vi "ResonanceAnalyzer_New_Guess_Frequency.vi"() -> ()   [LabVIEW 2014]
uses:
  <vilib>/imath/engines/lvmath/Plug In/_Char/NIMS_CH_character datatype.ctl
  <vilib>/imath/engines/lvmath2/RunTimeEngine/Managers/WorkSpace/UID Generator.vi
  <vilib>/imath/engines/lvmath2/RunTimeEngine/RunTimeType/NIMS_RunTimeType_From StrictType (excl LVString).vi
  <instcachedir>/0/NIMS_RunTimeType_From StrictType (excl LVString)_15A5391EEA9C4AACB9955AC755B83D29.lvgen/NIMS_RunTimeType_From StrictType (excl LVString)_15A5391EEA9C4AACB9955AC755B83D29_000.vi
  <vilib>/imath/engines/lvmath2/RunTimeEngine/LocalVariableDefStatement/MC_LocalVariableDefStatement_Display.vi
  <vilib>/imath/engines/lvmath2/RunTimeEngine/BuiltInFunctions/int32/NIMS_int32(real).vi
  <instcachedir>/0/NIMS_int32(real)_9F6AE75EF4BE45429513317A1C5A7040.lvgen/NIMS_int32(real)_9F6AE75EF4BE45429513317A1C5A7040_000.vi
  <vilib>/imath/engines/lvmath2/RunTimeEngine/BuiltInFunctions/linramp/NIMS_linramp.vi
  <vilib>/imath/engines/lvmath2/RunTimeEngine/RangeToken/NIMS_Range_R2 - Integer.vi
  <instcachedir>/0/NIMS_Range_R2 - Integer_2D1304BAF97744E0A293025746CBADFC.lvgen/NIMS_Range_R2 - Integer_2D1304BAF97744E0A293025746CBADFC_000.vi
  <vilib>/imath/engines/lvmath2/RunTimeEngine/CommandStatement/MC_CommandStatement_break.vi
  <vilib>/imath/engines/lvmath2/RunTimeEngine/IndexRead/NIMS V(S).vi
  <instcachedir>/0/NIMS V(S)_0488751826AF41519A22953C041130DC.lvgen/NIMS V(S)_0488751826AF41519A22953C041130DC_000.vi
  <vilib>/imath/engines/lvmath2/RunTimeEngine/IndexReplace/NIMS V(S)=S.vi
  <instcachedir>/0/NIMS V(S)=S_2D52C4EC15D8415E870AEE69FB516CCA.lvgen/NIMS V(S)=S_2D52C4EC15D8415E870AEE69FB516CCA_001.vi
  <vilib>/imath/engines/lvmath2/RunTimeEngine/ErrorHandling/NIMS_Create Error From Enums.vi
  <vilib>/imath/engines/lvmath/Plug In/_Char/NIMS_CH_Character RV to String.vi
  <instcachedir>/0/NIMS V(S)_0488751826AF41519A22953C041130DC.lvgen/NIMS V(S)_0488751826AF41519A22953C041130DC_003.vi
  <vilib>/imath/engines/lvmath2/RunTimeEngine/BuiltInFunctions/random/NIMS_random.vi
  <vilib>/imath/engines/lvmath2/RunTimeEngine/IndexReplace/NIMS V(S)=M.vi
  <instcachedir>/0/NIMS V(S)=M_608EF2A6197B4B6A9CB600D58D177061.lvgen/NIMS V(S)=M_608EF2A6197B4B6A9CB600D58D177061_001.vi
  <vilib>/imathl/engines/lvmath/Functions/Error Handling/Create Error.vi
  <vilib>/imath/engines/lvmath2/RunTimeEngine/BuiltInFunctions/and/NIMS_and.vi
  <instcachedir>/0/NIMS_and_04EBB299D59649339AD86944E4B9B28A.lvgen/NIMS_and_04EBB299D59649339AD86944E4B9B28A_000.vi
  <vilib>/imath/engines/lvmath/Functions/Error Handling/MergeErrorsWrapper.vi
  <vilib>/imath/engines/lvmath2/RunTimeEngine/Managers/SymbolTable/Clear UID.vi
  <vilib>/imath/engines/lvmath2/RunTimeEngine/NodeEndStatement/NIMS_NodeEndStatement_Output.vi
  <instcachedir>/0/NIMS_NodeEndStatement_Output_53EC0D466D134D7ABD903AC30B43404B.lvgen/NIMS_NodeEndStatement_Output_53EC0D466D134D7ABD903AC30B43404B_001.vi
  <instcachedir>/0/NIMS_NodeEndStatement_Output_53EC0D466D134D7ABD903AC30B43404B.lvgen/NIMS_NodeEndStatement_Output_53EC0D466D134D7ABD903AC30B43404B_010.vi
  <instcachedir>/0/NIMS_NodeEndStatement_Output_53EC0D466D134D7ABD903AC30B43404B.lvgen/NIMS_NodeEndStatement_Output_53EC0D466D134D7ABD903AC30B43404B_000.vi
  <instcachedir>/0/NIMS_NodeEndStatement_Output_53EC0D466D134D7ABD903AC30B43404B.lvgen/NIMS_NodeEndStatement_Output_53EC0D466D134D7ABD903AC30B43404B_005.vi
  <vilib>/imath/engines/lvmath2/RunTimeEngine/ErrorHandling/NIMS_Finalize Error.vi
  <vilib>/Utility/file.llb/Read From Spreadsheet File (DBL).vi
  <vilib>/imath/engines/lvmath2/RunTimeEngine/BuiltInFunctions/length/NIMS_length(GV).vi
  <instcachedir>/0/NIMS_length(GV)_08A3D13377FD4E4B96F5795FBF3698FA.lvgen/NIMS_length(GV)_08A3D13377FD4E4B96F5795FBF3698FA_000.vi
  <vilib>/imath/engines/lvmath2/RunTimeEngine/CommandStatement/NIMS_CommandStatement_MaskErr.vi
  <vilib>/imath/engines/lvmath2/RunTimeEngine/IndexRead/NIMS V(R2).vi
  <instcachedir>/0/NIMS V(R2)_C76619605A0E4E9F8B2FA9389712AC47.lvgen/NIMS V(R2)_C76619605A0E4E9F8B2FA9389712AC47_000.vi
  <vilib>/imath/engines/lvmath2/RunTimeEngine/Managers/SymbolTable/NIMS_WorkSpace.lvlib
panel:
  out "Non Lin Coefficients \n(Amp, Q fac, Center Freq)":dbl[](array[numeric])=[0.9672955512809506, 30.561485188767545, 656.7106190217593]
  out "residual":dynamicdata(graph)=[{"t0"=timestamp(0 s since 1904-01-01), "dt"=1.0, "Y"=[0.07958709642884196, 0.07429738045033185, 0.06826454630121676, 0.06261472934286921, 0.057591643274513576, 0.0524474377042822, 0.047364567198434376, 0.042486542348286, 0.0365475727577467, 0.02044337167913446, 0.015886366673806218, 0.002935673745636913, -0.010053830981330003, -0.023445458040964817, -0.04173930881285659, -0.049719042073960384, -0.018270334136156308, 0.010953780688973347, -0.005134983354591394, 0.009984081331178007, 0.032515930790111836, 0.01889369886358072, -0.03846899246991342, -0.045912443710329875, -0.03504278931549515, -0.024843357422279555, -0.018696932243340847, -0.012384162377026053, -0.006102276238951432, -0.0018255106598022153, 0.0035964852090220323, 0.007119092735802274, 0.012038929869804177], "attributes"=variant("NI_ChannelName"=variant(string "Residual"))}]
  out "Fit graph using coefficients":dynamicdata(graph)=[{"t0"=timestamp(0 s since 1904-01-01), "dt"=1.0, "Y"=[0.1295387978616468, 0.13721067023375874, 0.1457679401660022, 0.15537147781993743, 0.16622287352768353, 0.17857787895912505, 0.19276537754570408, 0.20921461245920156, 0.22849494645689253, 0.2513749070845742, 0.27891115728099847, 0.3125836541052877, 0.3544992932451337, 0.40768305317313946, 0.47641661786398076, 0.5662742095712869, 0.6822226232044952, 0.8533151124636015, 0.9552327939175806, 0.9461277661604174, 0.8357946509560049, 0.7011866250740231, 0.5852872341710728, 0.4949274767019172, 0.42567449552205106, 0.37206607131075253, 0.3298228761931464, 0.2959005518225358, 0.2681728686864641, 0.24514473245545426, 0.22574838621510776, 0.2092073116267047, 0.19494638542457107], "attributes"=variant("NI_ChannelName"=variant(string "Best fit"))}]
  out "Results":T1={"Q 2"=26.36, "Amp"=659.0, "Max Frequency"=0.9561118474915954}
  out "newFreq vs newAmp":cluster{"Freq":dbl[], "Amp":dbl[]}(graph)={"Freq"=[582.0, 586.0, 590.0, 594.0, 598.0, 602.0, 606.0, 610.0, 614.0, 618.0, 622.0, 626.0, 630.0, 634.0, 638.0, 642.0, 646.0, 651.0, 655.0, 659.0, 663.0, 667.0, 671.0, 675.0, 679.0, 683.0, 687.0, 691.0, 695.0, 699.0, 703.0, 707.0, 711.0], "Amp"=[0.20912589429048875, 0.2115080506840906, 0.21403248646721895, 0.21798620716280664, 0.2238145168021971, 0.23102531666340725, 0.24012994474413846, 0.25170115480748756, 0.2650425192146392, 0.2718182787637087, 0.2947975239548047, 0.3155193278509246, 0.3444454622638037, 0.38423759513217465, 0.43467730905112417, 0.5165551674973266, 0.6639522890683389, 0.8642688931525748, 0.9500978105629893, 0.9561118474915954, 0.8683105817461167, 0.7200803239376038, 0.5468182417011593, 0.44901503299158735, 0.3906317062065559, 0.347222713888473, 0.31112594394980553, 0.2835163894455097, 0.2620705924475127, 0.24331922179565205, 0.2293448714241298, 0.21632640436250697, 0.20698531529437525]}
  in  "Tab Control":enum32{"Simulation", "Experiment"}(tab)=enum."Experiment"
  in  "Center Frequency":dbl=600.0
  in  "Q":dbl=10.0
  in  "Start Frequency":dbl=400.0
  in  "End Frequency":dbl=800.0
  in  "df":dbl=5.0
  in  "Noise Level":dbl=0.003
  in  "Path":path=path "C:/Users/Jose/Documents/GitHub/week5/output2.txt"
  out "Freq and Gain Array":dbl[][](array[numeric])=[[400.0, 404.0, 408.0, 412.0, 416.0, 420.0, 424.0, 428.0, 432.0, 436.0, 440.0, 444.0, 448.0, 453.0, 457.0, 461.0, 465.0, 469.0, 473.0, 477.0, 481.0, 485.0, 489.0, 493.0, 497.0, 501.0, 505.0, 509.0, 513.0, 517.0, 521.0, 525.0, 529.0, 533.0, 537.0, 541.0, 545.0, 549.0, 554.0, 558.0, 562.0, 566.0, 570.0, 574.0, 578.0, 582.0, 586.0, 590.0, 594.0, 598.0, 602.0, 606.0, 610.0, 614.0, 618.0, 622.0, 626.0, 630.0, 634.0, 638.0, 642.0, 646.0, 651.0, 655.0, 659.0, 663.0, 667.0, 671.0, 675.0, 679.0, 683.0, 687.0, 691.0, 695.0, 699.0, 703.0, 707.0, 711.0, 715.0, 719.0, 723.0, 727.0, 731.0, 735.0, 739.0, 743.0, 747.0, 752.0, 756.0, 760.0, 764.0, 768.0, 772.0, 776.0, 780.0, 784.0, 788.0, 792.0, 796.0, 800.0], [-24.4709636621, -24.4900748326, -24.4321788401, -24.2882584883, -24.1019958302, -23.8592363876, -23.5767399504, -23.2699908646, -22.8946294875, -22.4045856715, -21.9111326853, -21.3295699884, -20.6610356502, -19.7008786093, -18.8234466029, -17.8330451216, -16.7094404547, -15.437484113, -13.7456060876, -11.8131615054, -9.8202094575, -8.2582107193, -7.7103161805, -8.2831973757, -9.4931334235, -11.4908968731, -13.3965570005, -14.9159357678, -16.131014729, -17.1374803263, -18.0639114173, -18.8469467487, -19.5518156394, -20.1377453264, -20.6596658267, -21.0994070544, -21.4760072311, -21.8051689199, -22.1344635319, -22.2543824181, -22.3980347688, -22.5619692766, -22.6441488194, -22.6526797483, -22.6288554102, -22.579660239, -22.4663939708, -22.3477465012, -22.1647066865, -21.900848007, -21.5837515908, -21.1972224629, -20.7265996938, -20.2101219656, -19.957687093, -19.1461369833, -18.4668251842, -17.5896669145, -16.4964136097, -15.2629852201, -13.5372036643, -11.0269216646, -8.3901852023, -7.4433752176, -7.3802755805, -8.3435299581, -10.2153969273, -12.9678599442, -14.9384609131, -16.3313727131, -17.5093605871, -18.6070466487, -19.5363252695, -20.3228855525, -21.0652820837, -21.656756001, -22.2411406116, -22.682546094, -23.1152710931, -23.4529459433, -23.7298559839, -23.9928500485, -24.170191316, -24.3014920023, -24.3954415293, -24.4316723757, -24.40625142, -24.2980363733, -24.1641378595, -24.0310090608, -23.7487352036, -23.4430503174, -23.0128990056, -22.6630698594, -22.0319754804, -21.4272021732, -20.7651149268, -19.7463173671, -18.8460529118, -17.674687366]] format="%0.3f"
  out "max":dbl=0.9561118474915954
  out "min":dbl=0.17275855369208631
  # "NOTE: x scale is in Time instead of Frequency"
  # "Note: accuracy is inversly proportional to P_in"
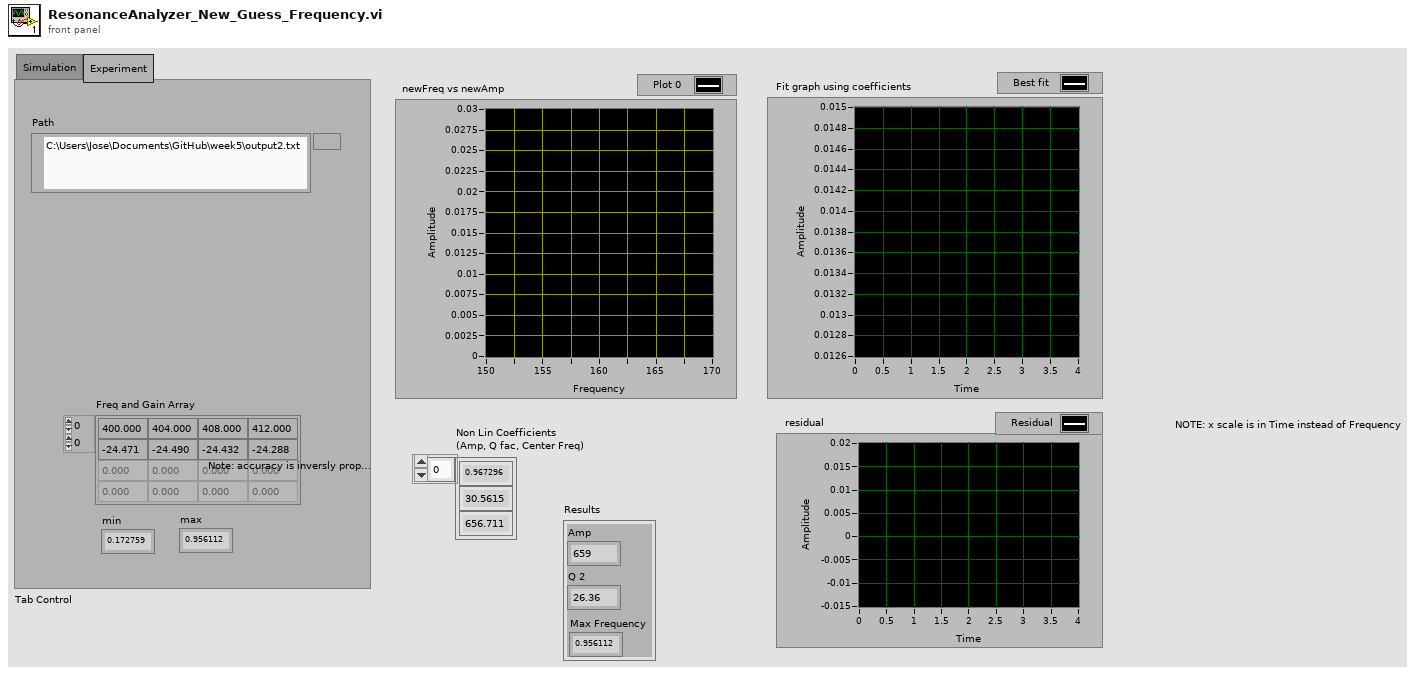
[diagram p1: front panel]
types:
  T1 = cluster{"Q 2":dbl, "Amp":dbl, "Max Frequency":dbl}
  T2 = typedef "NIMS_CH_character datatype.ctl" = cluster{"Numeric":u8}
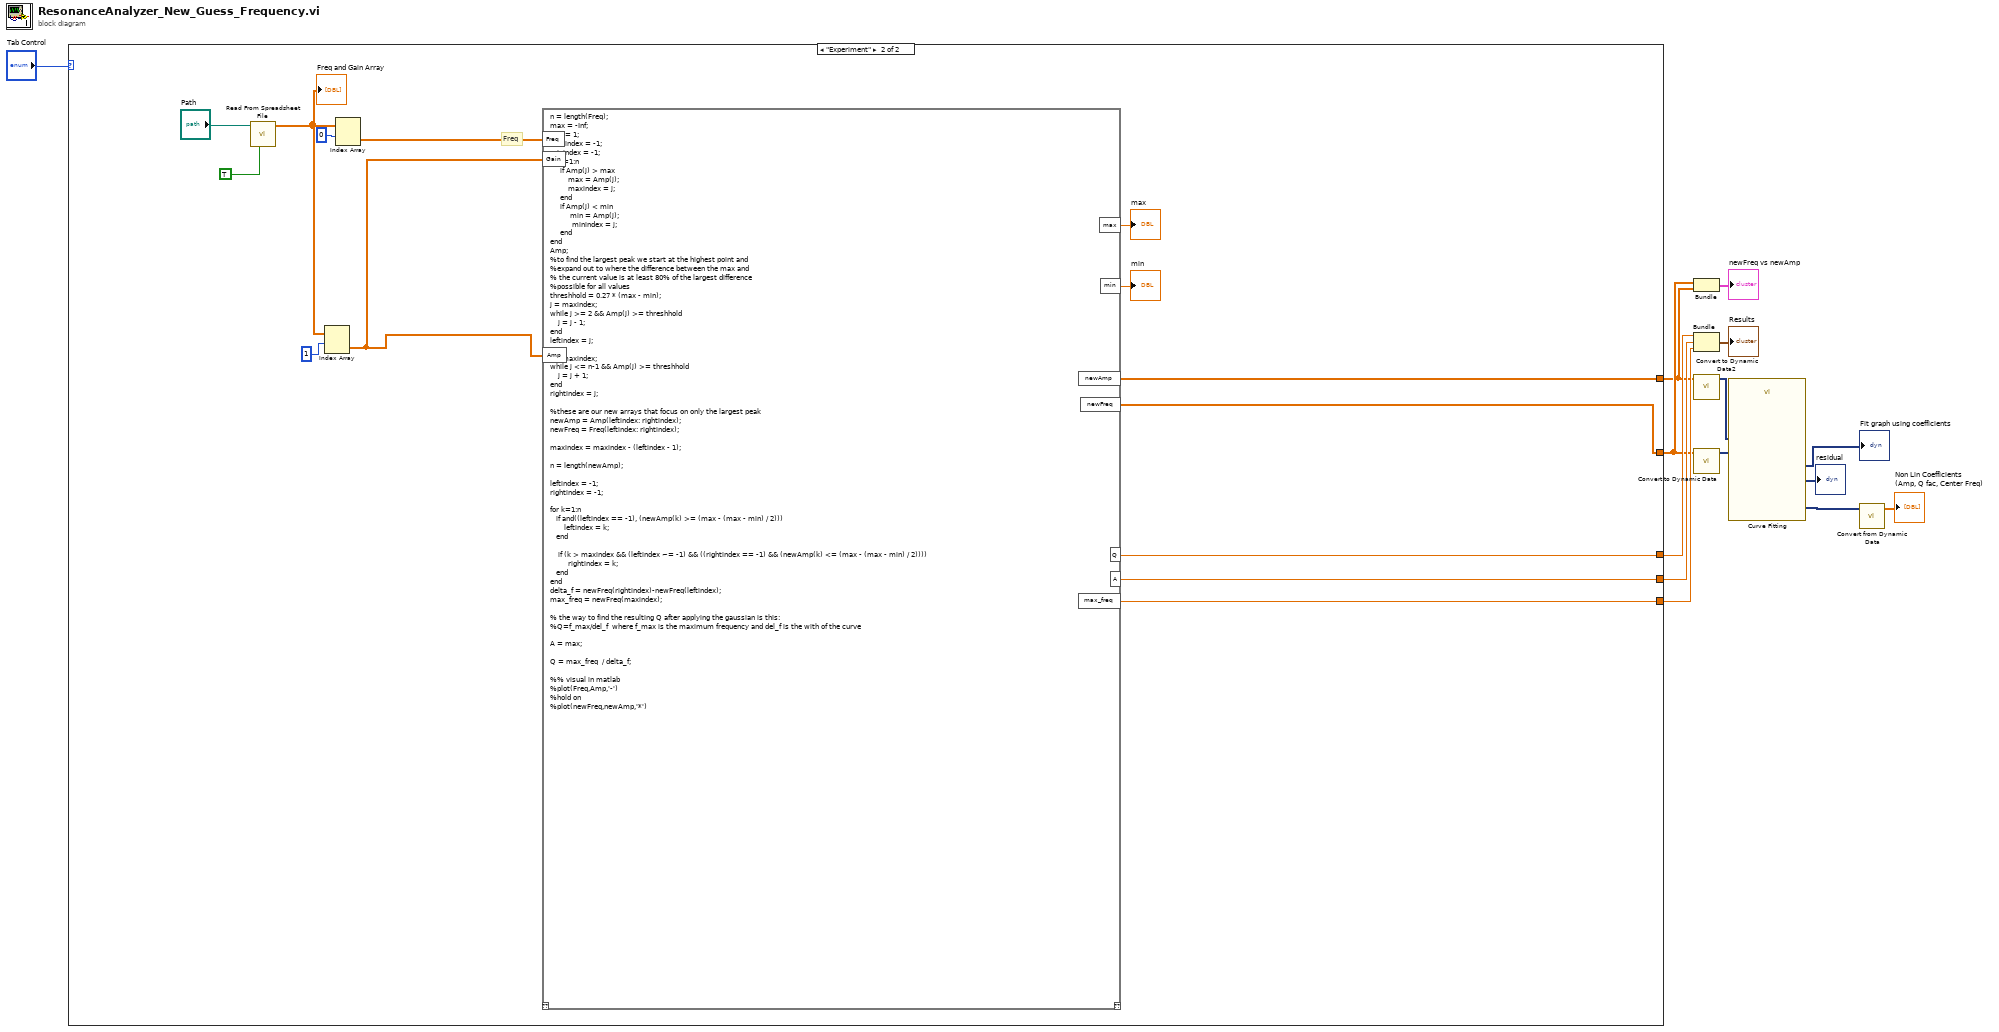
[diagram p0: block diagram]
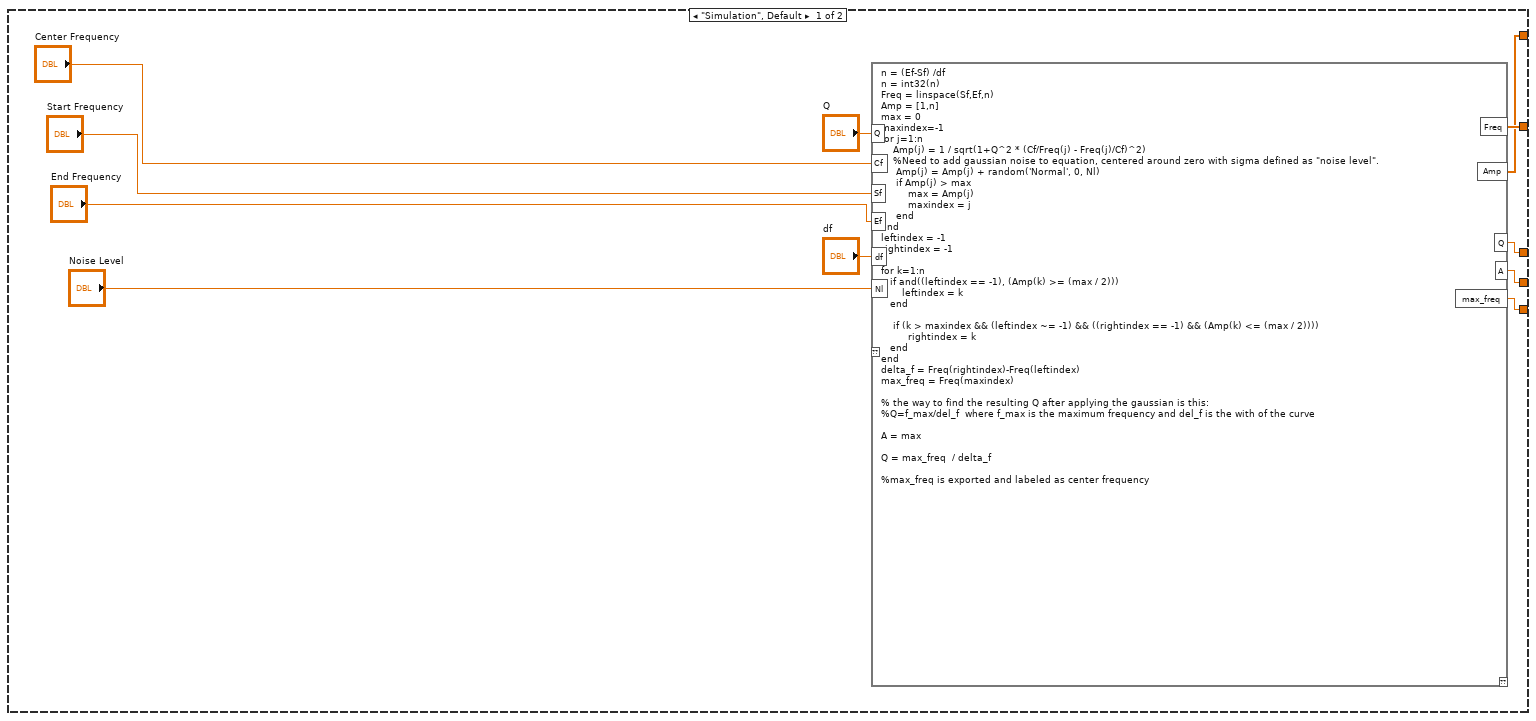
[diagram p2: hidden frame]
diagram:
  n1 = case shown="\"Experiment\"" "Tab Control" {
    tunnel: [w19 w675] -> w8
    tunnel: [w18 w676] -> w5
    tunnel: [w17 w674] -> w12
    tunnel: [w16 w673] -> w11
    tunnel: [w15 w672] -> w10
    frame "Simulation", Default {
      n2 = mathscript code="n = (Ef-Sf) /df\nn = int32(n)\nFreq = linspace(Sf,Ef,n)\nAmp = [1,n]\nmax = 0\nmaxindex=-1\nfor j=1:n\n    Amp(j) = 1 / sqrt(1+Q^2 * (Cf/Freq(j) - Freq(j)/Cf)^2)\n    %Need to add gaussian noise to equation, centered around zero with sigma defined as \"noise level\".\n     Amp(j) = Amp(j) + random('Normal', 0, Nl)\n     if Amp(j) > max\n         max = Amp(j)\n         maxindex = j\n     end\nend\nleftindex = -1\nrightindex = -1\n\nfor k=1:n\n   if and((leftindex == -1), (Amp(k) >= (max / 2)))\n       leftindex = k\n   end\n\n    if (k > maxindex && (leftindex ~= -1) && ((rightindex == -1) && (Amp(k) <= (max / 2))))\n         rightindex = k\n   end\nend\ndelta_f = Freq(rightindex)-Freq(leftindex)\nmax_freq = Freq(maxindex)\n\n% the way to find the resulting Q after applying the gaussian is this:\n%Q=f_max/del_f  where f_max is the maximum frequency and del_f is the with of the curve \n\nA = max\n\nQ = max_freq  / delta_f\n\n%max_freq is exported and labeled as center frequency"("Q"="Q", "Cf"="Center Frequency", "Sf"="Start Frequency", "Ef"="End Frequency", "df"="df", "Nl"="Noise Level") -> ("Freq"=w19:dbl[], "Amp"=w18:cdb[], "Q"=w17:dbl, "A"=w16:cdb, "max_freq"=w15:dbl)  [unwired: 1 in, 1 out]
    }
    frame "Experiment" {
      # "Freq"
      n3 = call-poly <vilib>:"Read From Spreadsheet File.vi"("transpose (no:F)"=TRUE, "file path (dialog if empty)"="Path") -> ("all rows"=w681:dbl[][])  [unwired: 5 in, 4 out]
      "Freq and Gain Array" <- w681
      n4 = Index Array(array=w681, index (row)=1) -> (element=w671:dbl[])  [unwired: 1 in]
      n5 = Index Array(array=w681, index (row)=0) -> (element=w679:dbl[])  [unwired: 1 in]
      n6 = mathscript code="n = length(Freq);\nmax = -Inf;\nmin = 1;\nmaxindex = -1;\nminindex = -1;\nfor j=1:n\n     if Amp(j) > max\n         max = Amp(j);\n         maxindex = j;\n     end\n     if Amp(j) < min\n          min = Amp(j);\n           minindex = j;\n     end\nend\nAmp;\n%to find the largest peak we start at the highest point and\n%expand out to where the difference between the max and \n% the current value is at least 80% of the largest difference \n%possible for all values \nthreshhold = 0.27 * (max - min);\nj = maxindex;\nwhile j >= 2 && Amp(j) >= threshhold\n    j = j - 1;\nend\nleftindex = j;\n\nj = maxindex;\nwhile j <= n-1 && Amp(j) >= threshhold\n    j = j + 1;\nend\nrightindex = j;\n\n%these are our new arrays that focus on only the largest peak\nnewAmp = Amp(leftindex: rightindex);\nnewFreq = Freq(leftindex: rightindex);\n\nmaxindex = maxindex - (leftindex - 1);\n\nn = length(newAmp);\n\nleftindex = -1;\nrightindex = -1;\n\nfor k=1:n\n   if and((leftindex == -1), (newAmp(k) >= (max - (max - min) / 2)))\n       leftindex = k;\n   end\n\n    if (k > maxindex && (leftindex ~= -1) && ((rightindex == -1) && (newAmp(k) <= (max - (max - min) / 2))))\n         rightindex = k;\n   end\nend\ndelta_f = newFreq(rightindex)-newFreq(leftindex);\nmax_freq = newFreq(maxindex);\n\n% the way to find the resulting Q after applying the gaussian is this:\n%Q=f_max/del_f  where f_max is the maximum frequency and del_f is the with of the curve \n\nA = max;\n\nQ = max_freq  / delta_f;\n\n%% visual in matlab\n%plot(Freq,Amp,'-')\n%hold on\n%plot(newFreq,newAmp,'*')"("Freq"=w679, "Gain"=w671, "Amp"=w671) -> ("max"=→"max":dbl, "min"=→"min":dbl, "newAmp"=w676:dbl[], "newFreq"=w675:dbl[], "Q"=w674:dbl, "A"=w673:dbl, "max_freq"=w672:dbl)  [unwired: 1 in, 1 out]
    }
  }
  n7 = Bundle("newFreq"=w8, "Amp"=w5) -> (→"newFreq vs newAmp":cluster{"newFreq":dbl[], "Amp":cdb[]})  [unwired: 1 in]
  n8 = Bundle("Q"=w12, "A"=w11, "max_freq"=w10) -> (→"Results":cluster{"Q":dbl, "A":cdb, "max_freq":dbl})  [unwired: 1 in]
  n9 = call "Convert to Dynamic Data2"("Array"=w5) -> ("Dynamic Data Type"=w6:dynamicdata)  [unwired: 3 in]
  n10 = call "Convert to Dynamic Data"("Array"=w8) -> ("Dynamic Data Type"=w7:dynamicdata)  [unwired: 3 in]
  n11 = call "Curve Fitting"("Locations"=w7, "Signals"=w6) -> ("residual"=→"residual":dynamicdata, "best fit"=→"Fit graph using coefficients":dynamicdata, "non-linear coefficients"=w4:dynamicdata)  [unwired: 5 in, 2 out]
  n12 = call "Convert from Dynamic Data"("Dynamic Data Type"=w4) -> ("Array"=→"Non Lin Coefficients \n(Amp, Q fac, Center Freq)":dbl[])  [unwired: 3 in]
